vi "Memory.Array.New.vi"(7 "allocation limit (2^31: 2GiB)":i64=2147483647 format="%08x bytes", 8 "error in (no error)":errorcluster, 9 "number of elements":u64, 10 "size of element":i64 format="%d bytes") -> (0 "error out":errorcluster, 3 "Array out":refnum<class "Memory.Array.Void.lvclass">)   [LabVIEW 2016, in "LabVIEW Memory Manager.lvlib" / "Memory.Array.Void.lvclass"]
uses:
  Memory.Array.Void.lvclass
  Pointer/Pointer.Void/Memory.Pointer.Void.lvclass/Memory.Pointer.Void.ctl
  Memory.Array.Void.lvclass/Memory.Array.Void.ctl
  Memory.Array.Set Pointer.vi
  Memory.Array.Set Element Size.vi
  Memory.Array.Set Number of Elements.vi
  Pointer/Pointer.Void/Methods/Memory.Pointer.New.vi
  Pointer/Pointer.Void/Methods/Memory.Pointer.Allocate.vi
  Pointer/Pointer.Void/Methods/Memory.Pointer.Set Address.vi
  Pointer/Pointer.Void/Methods/Memory.Pointer.Set Size.vi
  Pointer/Pointer.Void/Memory.Pointer.Void.lvclass
panel:
  out "allocated size":i64 format="%d bytes"
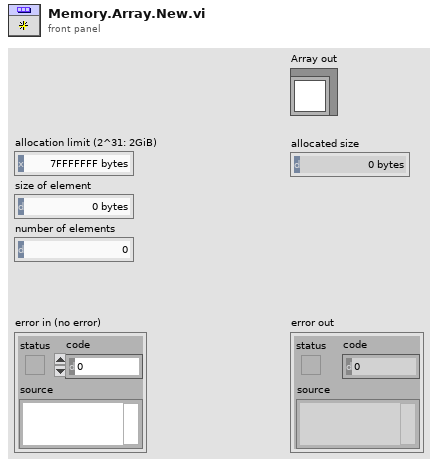
[diagram p1: front panel]
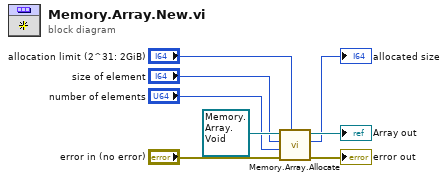
[diagram p0: block diagram]
diagram:
  n1 = call "Memory.Array.Allocate.vi"("allocation limit (2^31: 2GiB)"="allocation limit (2^31: 2GiB)", "error in (no error)"="error in (no error)", "number of elements"="number of elements", "size of element"="size of element", "Array in"=refnum<class "Memory.Array.Void.lvclass"> refnum) -> ("error out"=→"error out":errorcluster, "allocated size"=→"allocated size":i64, "Array out"=→"Array out":refnum<class "Memory.Array.Void.lvclass">)  [unwired: 4 in]
